vi "manual test UI.vi"(8 "error in (no error)":errorcluster caption="Fehler (Eingang, kein Fehler)", 11 "HF-Felder Eingang":refnum<class "HF-Felder.lvclass"> caption="DNL_LabVIEW Object in") -> (0 "error out":errorcluster caption="Fehler (Ausgang)", 1 "abbrechen out":bool, 2 "Parameters":u32[](array[numeric]), 3 "HF-Felder Ausgang":refnum<class "HF-Felder.lvclass"> caption="DNL_LabVIEW Object out")   [LabVIEW 2013, in "HF-Felder.lvclass"]
uses:
  HF-Felder.lvclass
  modulation.ctl
panel:
  in  "Testbeschreibung":string
  in  "Spannung (in V)":dbl=10.0 min=0.1 max=60.0 step=0.1
  in  "Stop Frequenz (in kHz)":u32=101 min=101 max=1000000
  in  "Start Frequenz (in kHz)":u32=100 min=100 max=1000000
  in  "Haltezeit (in s)":dbl=0.3 min=0.3 max=9999.9
  in  "Modulation":T1
  in  "abbrechen":bool
  in  "ok":bool
  # "Modulation"
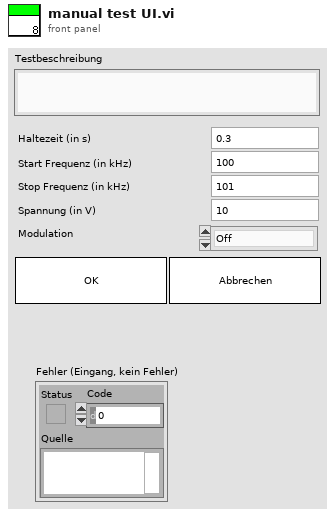
[diagram p1: front panel]
types:
  T1 = typedef "HF-Felder.lvclass/modulation.ctl" = enum16{"Off", "2Hz", "400Hz", "1kHz", "Pulse"}
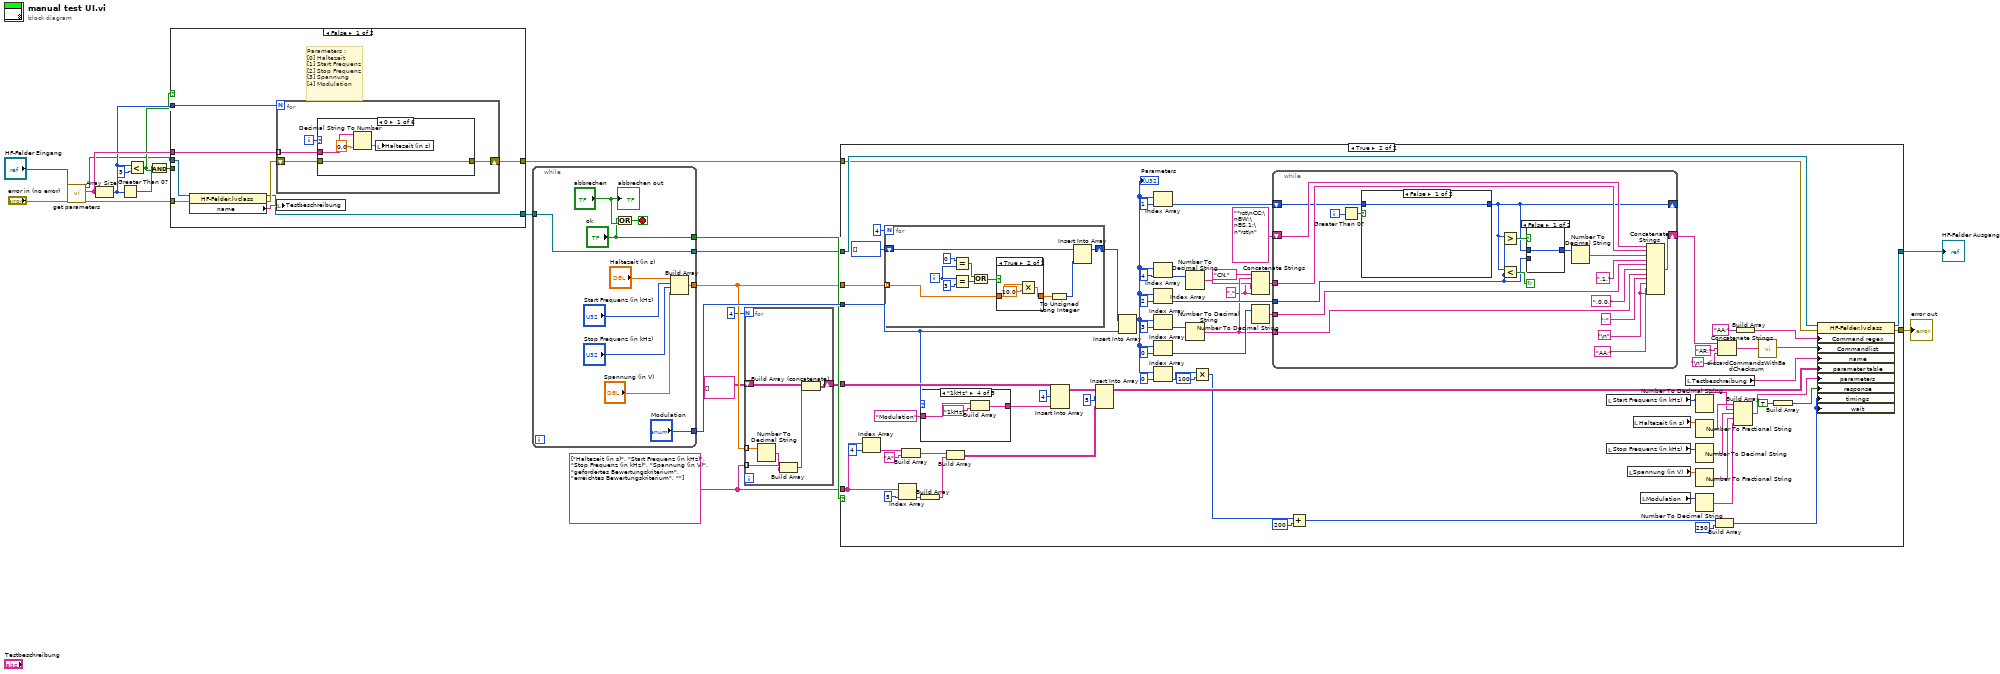
[diagram p0: block diagram]
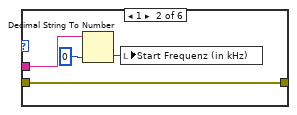
[diagram p2: hidden frame]
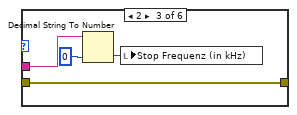
[diagram p3: hidden frame]
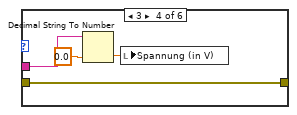
[diagram p4: hidden frame]
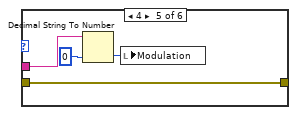
[diagram p5: hidden frame]
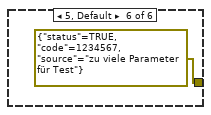
[diagram p6: hidden frame]
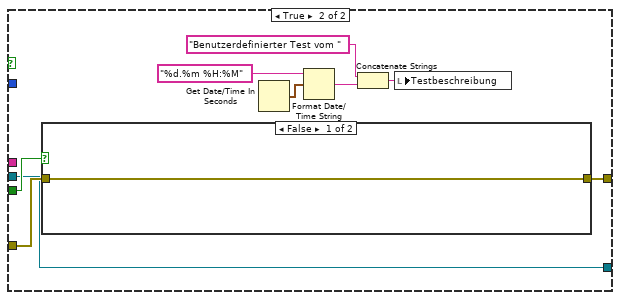
[diagram p7: hidden frame]
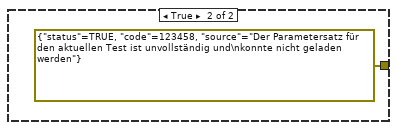
[diagram p8: hidden frame]
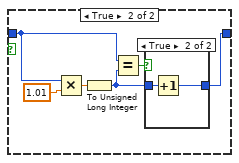
[diagram p10: hidden frame]
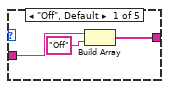
[diagram p14: hidden frame]
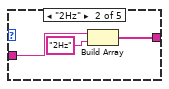
[diagram p15: hidden frame]
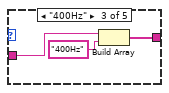
[diagram p16: hidden frame]
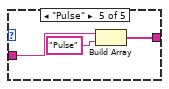
[diagram p17: hidden frame]
diagram:
  w13 = string[] ["Haltezeit (in s)", "Start Frequenz (in kHz)", "Stop Frequenz (in kHz)", "Spannung (in V)", "gefordertes Bewertungskriterium", "erreichtes Bewertungskriterium", ""]
  n1 = call-dynamic "get parameters.vi"("error in (no error)"="error in (no error)", "TestInterface (Eingang)"="HF-Felder Eingang") -> ("error out"=w10:errorcluster, "parameters"=w11:string[], "TestInterface (Ausgang)"=w3:refnum<class "HF-Felder.lvclass">)  [unwired: 7 in]
  n2 = Array Size(array=w11) -> (size(s)=w8:i32)
  n3 = Greater Than 0?(x=w8) -> (x > 0?=w7:bool)
  n4 = Less?(x=w8, y=5) -> (x < y?=w6:bool)
  n5 = And(x=w7, y=w6) -> (x .and. y?=w5:bool)
  n6 = case shown="False" w6 {
    tunnel: w8 -> [w30 _]
    tunnel: w11 -> [w29 _]
    tunnel: w10 -> [w26 w59]
    tunnel: [w28 w57] -> w1
    tunnel: w5 -> [_ w58]
    tunnel: w3 -> [w27 w56]
    tunnel: [w23 w56] -> w2
    frame False {
      # "Parameters :\n[0] Haltezeit\n[1] Start Frequenz\n[2] Stop Frequenz\n[3] Spannung\n[4] Modulation"
      n7 = property class="HF-Felder.lvclass"(reference=w27, error in=w26) -> (reference out=w23:refnum<class "HF-Felder.lvclass">, error out=w25:errorcluster, "name"=w24:string)
      n8 = for {
        N: w30 -> [_]
        tunnel: w29 -> [w33] mode=indexing
        shift-right: [w32] -> w28
        shift-left: w25 -> [w31]
        i -> [w34]
        n9 = case shown="0" w34 {
          tunnel: w33 -> [w38 w40 w44 w48 w52 _]
          tunnel: w31 -> [w35 w39 w43 w47 w51 _]
          tunnel: [w35 w39 w43 w47 w51 errorcluster {"status"=TRUE, "code"=1234567, "source"="zu viele Parameter für Test"} ("error constant")] -> w32
          frame 0 {
            n10 = Decimal String To Number(string=w38, default (0L)=0.0 ("default (0 I32)")) -> (number=w37:dbl)  [unwired: 1 in, 1 out]
            n11 = local write "Haltezeit (in s)"(w37) -> ()
          }
          frame 1 {
            n12 = Decimal String To Number(string=w40, default (0L)=u32 0 ("default (0 I32)")) -> (number=w41:u32)  [unwired: 1 in, 1 out]
            n13 = local write "Start Frequenz (in kHz)"(w41) -> ()
          }
          frame 2 {
            n14 = Decimal String To Number(string=w44, default (0L)=u32 0 ("default (0 I32)")) -> (number=w45:u32)  [unwired: 1 in, 1 out]
            n15 = local write "Stop Frequenz (in kHz)"(w45) -> ()
          }
          frame 3 {
            n16 = Decimal String To Number(string=w48, default (0L)=0.0 ("default (0 I32)")) -> (number=w49:dbl)  [unwired: 1 in, 1 out]
            n17 = local write "Spannung (in V)"(w49) -> ()
          }
          frame 4 {
            n18 = Decimal String To Number(string=w52, default (0L)=u32 0 ("default (0 I32)")) -> (number=w53:u32)  [unwired: 1 in, 1 out]
            n19 = local write "Modulation"(w53) -> ()
          }
          frame 5, Default {
          }
        }
      }
      n20 = local write "Testbeschreibung"(w24) -> ()
    }
    frame True {
      n21 = case shown="False" w58 {
        tunnel: w59 -> [w65 _]
        tunnel: [w65 errorcluster {"status"=TRUE, "code"=123458, "source"="Der Parametersatz für den aktuellen Test ist unvollständig und\nkonnte nicht geladen werden"} ("error constant")] -> w57
        frame False {
        }
        frame True {
        }
      }
      n22 = Get Date/Time In Seconds() -> (seconds since 1Jan1904=w64:timestamp)
      n23 = Format Date/Time String(time format string (%c)="%d.%m %H:%M" ("Zeitformatierungs-String (%c)"), seconds (now)=w64) -> (date/time string=w61:string)  [unwired: 1 in]
      n24 = Concatenate Strings("Benutzerdefinierter Test vom " ("name"), w61) -> (w60:string)
      n25 = local write "Testbeschreibung"(w60) -> ()
    }
  }
  n26 = while {
    tunnel: [w74] -> w20
    tunnel: w2 -> [w74]
    tunnel: ["Modulation"] -> w22
    tunnel: ["ok"] -> w21
    tunnel: [w67] -> w17
    stop <- w75 stop-if-true
    n27 = Or(x="ok", y="abbrechen") -> (x .or. y?=w75:bool)
    n28 = Build Array("Haltezeit (in s)", "Start Frequenz (in kHz)", "Stop Frequenz (in kHz)", "Spannung (in V)") -> (w67:dbl[])
    "abbrechen out" <- "abbrechen"
  }
  n29 = for {
    N: 4 -> [_]
    tunnel: w17 -> [w81] mode=indexing
    tunnel: w13 -> [w82] mode=indexing
    shift-right: [w77] -> w14
    shift-left: string[][] [] -> [w79]
    n30 = Number To Decimal String(number=w81) -> (decimal integer string=w80:string)  [unwired: 1 in]
    n31 = Build Array(w82, w80) -> (w78:string[])
    n32 = Build Array (concatenate)(w79, w78) -> (w77:string[][])
  }
  n33 = case shown="True" w21 {
    tunnel: w22 -> [_ w152]
    tunnel: w14 -> [_ w154]
    tunnel: w20 -> [w84 w136]
    tunnel: [w84 w135] -> w19
    tunnel: w1 -> [w83 w134]
    tunnel: [w83 w133] -> w18
    tunnel: w17 -> [_ w148]
    tunnel: w13 -> [_ w140]
    frame False {
    }
    frame True {
      w105 = "," ("String")
      n34 = Index Array(array=w140, index=4 ("Index")) -> (element=w144:string)
      n35 = for {
        N: 4 -> [_]
        shift-right: [w192] -> w151
        shift-left: u32[] [] -> [w193]
        tunnel: w148 -> [w188] mode=indexing
        i -> [w189]
        n36 = Equal?(x=u32 0, y=w189) -> (x = y?=w198:bool)
        n37 = Equal?(x=w189, y=u32 3) -> (x = y?=w197:bool)
        n38 = Or(x=w198, y=w197) -> (x .or. y?=w194:bool)
        n39 = case shown="True" w194 {
          tunnel: w188 -> [w199 w202]
          tunnel: [w199 w200] -> w191
          frame False {
          }
          frame True {
            n40 = Multiply(x=w202, y=10.0) -> (x*y=w200:dbl)
          }
        }
        n41 = To Unsigned Long Integer(number=w191) -> (unsigned 32bit integer=w190:u32)
        n42 = Insert Into Array(array=w193, new element=w190) -> (w192:u32[])  [unwired: 1 in]
      }
      n43 = Index Array(array=w140, index=5 ("Index")) -> (element=w143:string)
      n44 = Build Array(w144, "A" ("Element")) -> (w146:string[])
      n45 = case shown="\"1kHz\"" w152 {
        tunnel: "Modulation" -> [w205 w207 w210 w213 w216]
        tunnel: [w203 w206 w209 w212 w215] -> w155
        frame "Off", Default {
          n46 = Build Array(w205, "Off" ("Element")) -> (w203:string[])
        }
        frame "2Hz" {
          n47 = Build Array(w207, "2Hz" ("Element")) -> (w206:string[])
        }
        frame "400Hz" {
          n48 = Build Array(w210, "400Hz" ("Element")) -> (w209:string[])
        }
        frame "1kHz" {
          n49 = Build Array(w213, "1kHz" ("Element")) -> (w212:string[])
        }
        frame "Pulse" {
          n50 = Build Array(w216, "Pulse" ("Element")) -> (w215:string[])
        }
      }
      n51 = Build Array(w143) -> (w147:string[])
      n52 = Build Array(w146, w147) -> (w137:string[][])
      n53 = Insert Into Array(array=w154, index (row)=4, new element=w155) -> (w138:string[][])  [unwired: 1 in]
      n54 = Insert Into Array(array=w138, index (row)=5 ("Index (Zeile)"), new element=w137) -> (w123:string[][])  [unwired: 1 in]
      n55 = Insert Into Array(array=w151, new element=w152) -> (w94:u32[])  [unwired: 1 in]
      "Parameters" <- w94
      n56 = Index Array(array=w94, index=1) -> (element=w120:u32)
      n57 = Index Array(array=w94, index=4) -> (element=w107:u32)
      n58 = Index Array(array=w94, index=2) -> (element=w118:u32)
      n59 = Index Array(array=w94, index=3) -> (element=w116:u32)
      n60 = Index Array(array=w94, index=0) -> (element=w111:u32)
      n61 = Index Array(array=w94, index=0) -> (element=w97:u32)
      n62 = Number To Decimal String(number=w107) -> (decimal integer string=w106:string)  [unwired: 1 in]
      n63 = Number To Decimal String(number=w116) -> (decimal integer string=w109:string)  [unwired: 1 in]
      n64 = Multiply(x=w97, y=u32 100) -> (x*y=w99:u32)
      n65 = Concatenate Strings("CN,", w109, w105, w106, w105) -> (w114:string)
      n66 = Number To Decimal String(number=w111) -> (decimal integer string=w112:string)  [unwired: 1 in]
      n67 = while {
        shift-right: [w175] -> w104
        shift-left: "*rst\nCC;\nBW;\nBS,1;\n*rst\n" -> [w174]
        tunnel: w114 -> [w173]
        tunnel: w118 -> [w168]
        shift-right: [w167] -> _
        shift-left: w120 -> [w170]
        tunnel: w112 -> [w163]
        tunnel: w109 -> [w157]
        i -> [w159]
        stop <- w171 continue-if-true
        w160 = "\n"
        n68 = Greater Than 0?(x=w159) -> (x > 0?=w158:bool)
        n69 = case shown="False" w158 {
          tunnel: w170 -> [w176 w180]
          tunnel: [w176 w179] -> w167
          frame False {
          }
          frame True {
            n70 = Multiply(x=w180, y=1.01) -> (x*y=w178:dbl)
            n71 = To Unsigned Long Integer(number=w178) -> (unsigned 32bit integer=w182:u32)
            n72 = Equal?(x=w180, y=w182) -> (x = y?=w181:bool)
            n73 = case shown="True" w181 {
              tunnel: w182 -> [w183 w184]
              tunnel: [w183 w185] -> w179
              frame False {
              }
              frame True {
                n74 = Increment(x=w184) -> (x+1=w185:u32)
              }
            }
          }
        }
        n75 = Greater?(x=w167, y=w168) -> (0:w169:bool)
        n76 = Less?(x=w167, y=w168) -> (x < y?=w171:bool)
        n77 = case shown="False" w169 {
          tunnel: w168 -> [_ w187]
          tunnel: w167 -> [w186 _]
          tunnel: [w186 w187] -> w166
          frame False {
          }
          frame True {
          }
        }
        n78 = Number To Decimal String(number=w166) -> (decimal integer string=w172:string)  [unwired: 1 in]
        n79 = Concatenate Strings(w174, w173, w172, ",1," ("string"), w163, ",0,0," ("string"), w157, ";" ("string"), w160, "AA;", w160) -> (w175:string)
      }
      n80 = Add(x=w99, y=u32 200) -> (x+y=w101:u32)
      n81 = local read "Start Frequenz (in kHz)"() -> (w130:u32)
      n82 = local read "Stop Frequenz (in kHz)"() -> (w131:u32)
      n83 = local read "Spannung (in V)"() -> (w129:dbl)
      n84 = local read "Haltezeit (in s)"() -> (w128:dbl)
      n85 = local read "Modulation"() -> (w132:T1)
      n86 = local read "Testbeschreibung"() -> (w122:string)
      n87 = Number To Decimal String(number=w130) -> (decimal integer string=w87:string)  [unwired: 1 in]
      n88 = Number To Fractional String(number=w128) -> (F-format string=w88:string)  [unwired: 3 in]
      n89 = Number To Decimal String(number=w131) -> (decimal integer string=w127:string)  [unwired: 1 in]
      n90 = Number To Fractional String(number=w129) -> (F-format string=w126:string)  [unwired: 3 in]
      n91 = Number To Decimal String(number=w132) -> (decimal integer string=w125:string)  [unwired: 1 in]
      n92 = Build Array(w101, u32 250 ("element")) -> (w93:u32[])
      n93 = Concatenate Strings(w104, "AR;" ("string"), "\n") -> (w86:string)
      n94 = Build Array(w88, w87, w127, w126, w125) -> (w124:string[])
      n95 = Build Array("AA;") -> (w90:string[])
      n96 = call "discardCommandsWithBadChecksum.vi"("multi-line string"=w86) -> ("outputstring"=w85:string)  [unwired: 10 in]
      n97 = Build Array(TRUE) -> (w89:bool[])
      n98 = property class="HF-Felder.lvclass"(reference=w136, error in=w134, "Command regex"=w90, "Commandlist"=w85, "name"=w122, "parameter table"=w123, "parameters"=w124, "response"=w89, "timings"=w93, "wait"=w93) -> (reference out=w135:refnum<class "HF-Felder.lvclass">, error out=w133:errorcluster)
    }
  }
  "HF-Felder Ausgang" <- w19
  "error out" <- w18
